vi "ADC_config.vi"(1 "Inst_parameter":T1={"Kind"=0, "Strings"=["ADC", "", "V", "ADC0;ADC1", "V;V"], "uint64s"=[10, 2, 250000, 0, 100, 10106, 1000000], "Doubles"=[1.0], "DAQmx take out list"=[]}) -> (0 "Inst_parameter out":T1)   [LabVIEW 2013]
uses:
  <vilib>/DAQmx/create/channels.llb/DAQmx Create Channel (AI-Voltage-Basic).vi
panel:
  out "error out":errorcluster
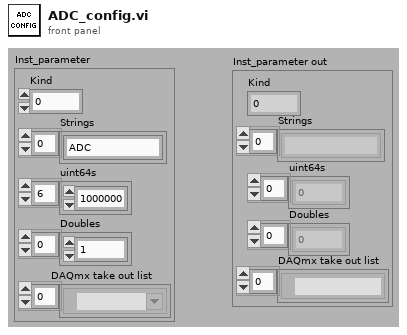
[diagram p1: front panel]
types:
  T1 = cluster{"Kind":u16, "Strings":string[], "uint64s":u64[], "Doubles":dbl[], "DAQmx take out list":refnum<k21>[]}
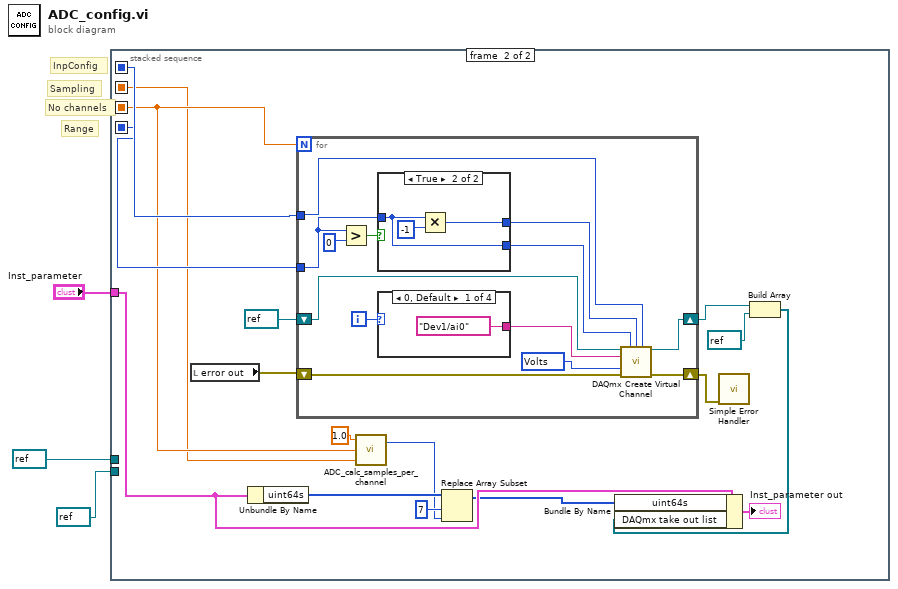
[diagram p0: block diagram]
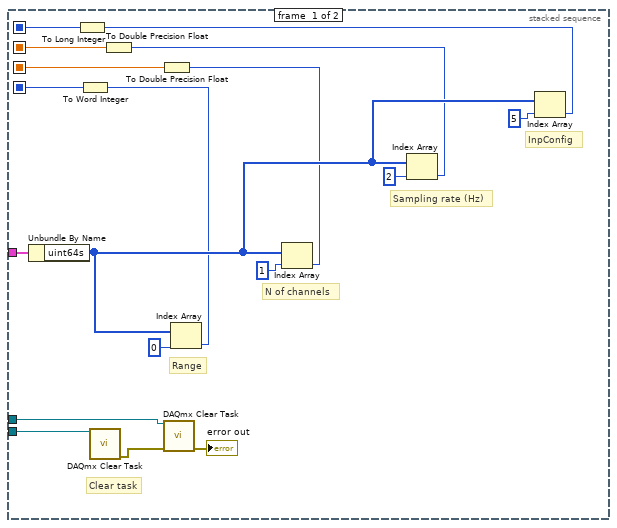
[diagram p2: hidden frame]
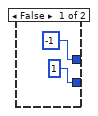
[diagram p3: hidden frame]
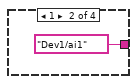
[diagram p4: hidden frame]
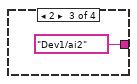
[diagram p5: hidden frame]
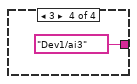
[diagram p6: hidden frame]
diagram:
  # "Range"
  # "No channels"
  # "Sampling"
  # "InpConfig"
  n1 = stacked-sequence {
    seq-local: [w8 _] -> [_ w37]
    seq-local: [w5 _] -> [_ w32]
    seq-local: [w7 _] -> [_ w33]
    seq-local: [w6 _] -> [_ w36]
    tunnel: refnum<k21> refnum ("internal clock") -> [w20 _]
    tunnel: refnum<k21> refnum ("task out in") -> [w19 _]
    tunnel: "Inst_parameter" -> [w18 w25]
    frame #0 {
      # "Range"
      # "N of channels"
      # "Sampling rate (Hz)"
      # "InpConfig"
      # "Clear task"
      n2 = Unbundle By Name(w18) -> ("uint64s"=w17:u64[])
      n3 = call <vilib>:"DAQmx Clear Task.vi"("task in"=w20) -> ("error out"=w21:errorcluster)  [unwired: 14 in]
      n4 = call <vilib>:"DAQmx Clear Task.vi"("task in"=w19, "error in"=w21) -> ("error out"=→"error out":errorcluster)  [unwired: 13 in]
      n5 = Index Array(array=w17, index=0) -> (element=w9:u64)
      n6 = To Word Integer(number=w9) -> (16bit integer=w6:i16)
      n7 = Index Array(array=w17, index=1) -> (element=w10:u64)
      n8 = To Double Precision Float(number=w10) -> (double precision float=w7:dbl)
      n9 = Index Array(array=w17, index=2) -> (element=w11:u64)
      n10 = To Double Precision Float(number=w11) -> (double precision float=w5:dbl)
      n11 = Index Array(array=w17, index=5) -> (element=w12:u64)
      n12 = To Long Integer(number=w12) -> (32bit integer=w8:i32)
    }
    frame #1 {
      n13 = local read "error out"() -> (w35:errorcluster)
      n14 = Unbundle By Name(w25) -> ("uint64s"=w28:u64[])
      n15 = for {
        N: w33 -> [_]
        shift-right: [w51] -> w29
        shift-left: refnum<k21> refnum ("task out") -> [w50]
        shift-right: [w47] -> w34
        shift-left: w35 -> [w46]
        tunnel: w36 -> [w43]
        tunnel: w37 -> [w39]
        i -> [w40]
        w48 = 10348 items=["Volts"=10348, "From Custom Scale"=10065] ("units")
        n16 = Greater?(x=w43, y=i16 0) -> (0:w44:bool)
        n17 = case shown="True" w44 {
          tunnel: w43 -> [_ w54]
          tunnel: [i16 -1 w55] -> w45
          tunnel: [i16 1 ("Range") w54] -> w41
          frame False {
          }
          frame True {
            n18 = Multiply(x=w54, y=i16 -1) -> (x*y=w55:i16)
          }
        }
        n19 = case shown="0, Default" w40 {
          tunnel: [tag "Dev1/ai0" ("physical channels") tag "Dev1/ai1" ("physical channels") tag "Dev1/ai2" ("physical channels") tag "Dev1/ai3" ("physical channels")] -> w49
          frame 0, Default {
          }
          frame 1 {
          }
          frame 2 {
          }
          frame 3 {
          }
        }
        n20 = call-poly <vilib>:"DAQmx Create Virtual Channel.vi"("task in"=w50, "maximum value"=w41, "minimum value"=w45, "input terminal configuration"=w39, "physical channels"=w49, "units"=w48, "error in"=w46) -> ("task out"=w51:refnum<k21>, "error out"=w47:errorcluster)  [unwired: 2 in, 5 out]
      }
      n21 = call "ADC_calc_samples_per_channel.vi"("Samplingrate"=w32, "Nchannel"=w33, "time per point (ms)"=1.0) -> ("samples to read"=w26:u32)  [unwired: 1 out]
      n22 = Replace Array Subset(array=w28, new element=w26, index=7) -> (w24:u64[])
      n23 = call <vilib>:"Simple Error Handler.vi"("error in (no error)"=w34) -> ()  [unwired: 4 in, 5 out]
      n24 = Build Array(w29, refnum<k21> refnum ("internal clock")) -> (w23:refnum<k21>[])
      n25 = Bundle By Name(cluster=w25, "uint64s"=w24, "DAQmx take out list"=w23) -> (→"Inst_parameter out":T1)
    }
  }
